vi "Save Serial Number - Serial.vi"(8 "error in":errorcluster, 9 "starting address":u16, 11 "Modbus master in":refnum<class "Modbus Master.lvclass">) -> (0 "error out":errorcluster, 2 "SN ok":bool, 3 "Modbus master out":refnum<class "Modbus Master.lvclass">, 4 "register values":u16[](array[numeric]), 5 "SN":i32[](array[numeric]))   [LabVIEW 2023]
uses:
  <vilib>/NI/Modbus Library/API/Master/Modbus Master.lvclass
  RS485/RS485.lvlib
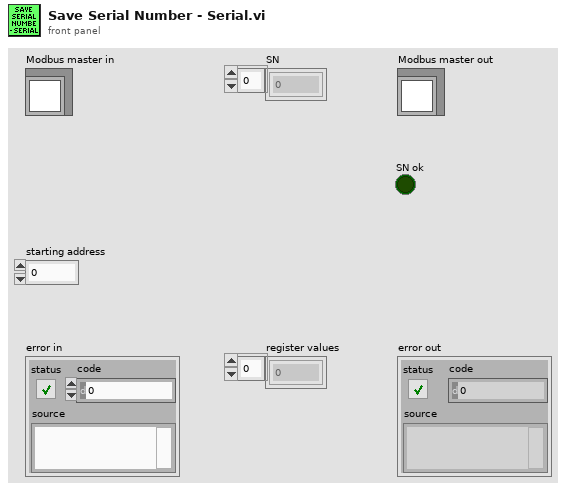
[diagram p1: front panel]
types:
  T1 = typedef "LVDateTimeRec.ctl" = cluster{"fractional second":dbl, "second":i32, "minute":i32, "hour":i32, "day of month":i32, "month":i32, "year":i32, "day of week":i32, "day of year":i32, "DST":i32}
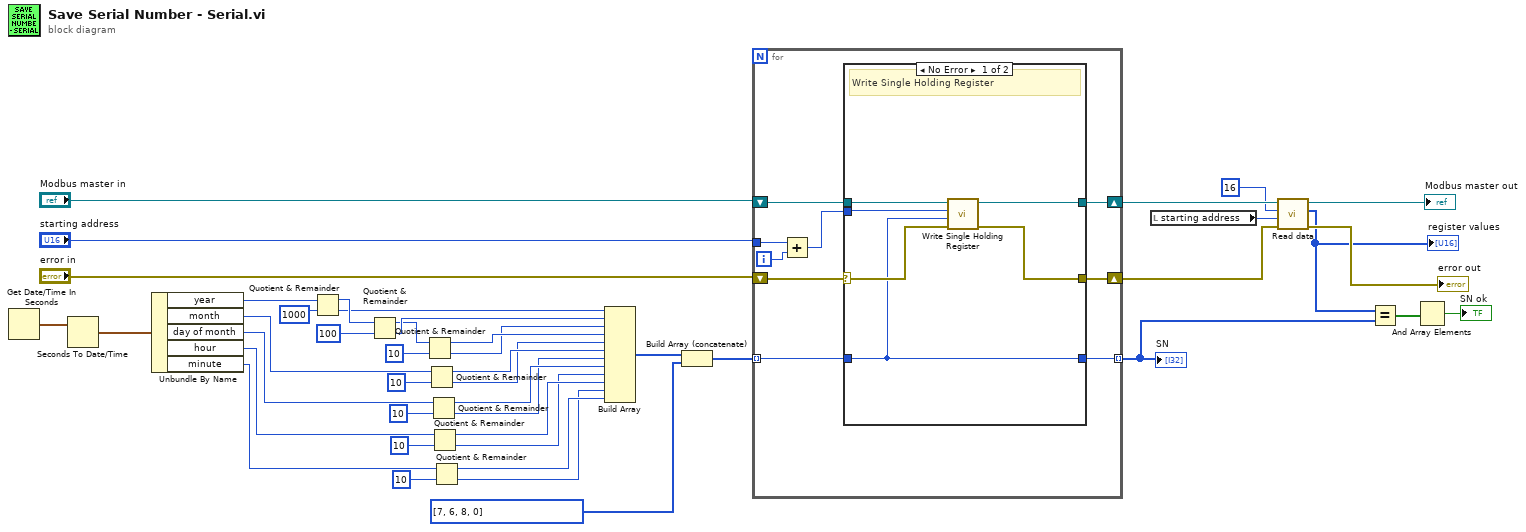
[diagram p0: block diagram]
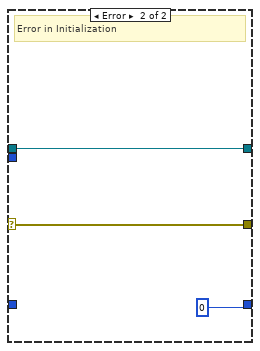
[diagram p2: hidden frame]
diagram:
  n1 = Get Date/Time In Seconds() -> (seconds since 1Jan1904=w41:timestamp)
  n2 = Seconds To Date/Time(time stamp (now)=w41) -> (date time rec=w40:T1)  [unwired: 1 in]
  n3 = Unbundle By Name(w40) -> ("year"=w39:i32, "month"=w28:i32, "day of month"=w24:i32, "hour"=w19:i32, "minute"=w16:i32)
  n4 = Quotient & Remainder(x=w39, y=1000) -> (x-y*floor(x/y)=w37:i32, floor(x/y)=w36:i32)
  n5 = Quotient & Remainder(x=w37, y=100) -> (x-y*floor(x/y)=w33:i32, floor(x/y)=w34:i32)
  n6 = Quotient & Remainder(x=w33, y=10) -> (x-y*floor(x/y)=w31:i32, floor(x/y)=w29:i32)
  n7 = Quotient & Remainder(x=w28, y=10) -> (x-y*floor(x/y)=w27:i32, floor(x/y)=w25:i32)
  n8 = Quotient & Remainder(x=w24, y=10) -> (x-y*floor(x/y)=w23:i32, floor(x/y)=w21:i32)
  n9 = Quotient & Remainder(x=w19, y=10) -> (x-y*floor(x/y)=w20:i32, floor(x/y)=w17:i32)
  n10 = Quotient & Remainder(x=w16, y=10) -> (x-y*floor(x/y)=w15:i32, floor(x/y)=w14:i32)
  n11 = Build Array(w36, w34, w29, w31, w25, w27, w21, w23, w17, w20, w14, w15) -> (w13:i32[])
  n12 = Build Array (concatenate)(w13, i32[] [7, 6, 8, 0] ("array")) -> (w11:i32[])
  n13 = for {
    tunnel: "starting address" -> [w49]
    shift-right: [w51] -> w10
    shift-left: "Modbus master in" -> [w53]
    shift-right: [w50] -> w6
    shift-left: "error in" -> [w52]
    tunnel: w11 -> [w46] mode=indexing
    tunnel: [w45] -> w4 mode=indexing
    i -> [w48]
    n14 = Add(x=w49, y=w48) -> (x+y=w47:i32)
    n15 = case shown="No Error" w52 {
      selector: w52 -> [w57 w61]
      tunnel: w53 -> [w59 w62]
      tunnel: [w58 w62] -> w51
      tunnel: [w56 w61] -> w50
      tunnel: w47 -> [w55 _]
      tunnel: w46 -> [w54 _]
      tunnel: [w54 0] -> w45
      frame No Error {
        # "Write Single Holding Register"
        n16 = call-dynamic "Write Single Holding Register.vi"("error in"=w57, "register to write"=w54, "address"=w55, "Modbus master in"=w59) -> ("error out"=w56:errorcluster, "Modbus master out"=w58:refnum<class "Modbus Master.lvclass">)  [unwired: 6 in]
      }
      frame Error {
        # "Error in Initialization"
      }
    }
  }
  "SN" <- w4
  n17 = local read "starting address"() -> (w7:u16)
  n18 = call "Read data.vi"("error in"=w6, "starting address"=w7, "number of inputs"=u16 16, "Modbus master in"=w10) -> ("error out"=→"error out":errorcluster, "register values"=w3:u16[], "Modbus master out"=→"Modbus master out":refnum<class "Modbus Master.lvclass">)  [unwired: 5 in]
  "register values" <- w3
  n19 = Equal?(x=w3, y=w4) -> (x = y?=w2:bool[])
  n20 = And Array Elements(Boolean array=w2) -> (logical AND=→"SN ok":bool)
